vi "Main.vi"() -> ()   [LabVIEW 2016]
uses:
  <vilib>/Instr/_visa.llb/VISA Open Access Mode.ctl
  <vilib>/Instr/_visa.llb/VISA Configure Serial Port (Instr).vi
panel:
  in  "Tab Control":enum32{"Main Program", "Calibration"}(tab)
  in  "Sampling rate (sample/s)":dbl=10.0
  out "Waveform Chart":cluster{u8, u8, u8, u8, u8, u8, u8, u8}(graph)
  in  "Current set (mA)":u16[](array[numeric])
  in  "update curr":bool
  out "Thermometer":i8(slide) scale=10.0..130.0
  out "Temp °C":i8
  in  "VISA resource name":refnum<visa-resource-name>
  in  "relay_1":bool
  in  "relay_2":bool
  in  "relay_3":bool
  in  "relay_4":bool
  in  "relay_5":bool
  in  "relay_6":bool
  in  "relay_7":bool
  out "connected?":bool
  in  "Ch1":bool
  in  "Ch2":bool
  in  "Ch3":bool
  in  "Ch4":bool
  in  "Ch5":bool
  in  "Ch6":bool
  in  "Ch7":bool
  in  "Ch8":bool
  in  "active_ch 1":bool
  in  "active_ch 2":bool
  in  "active_ch 3":bool
  in  "active_ch 4":bool
  in  "active_ch 5":bool
  in  "active_ch 6":bool
  in  "active_ch 7":bool
  in  "active_ch 8":bool
  in  "START":bool
  in  "stop 2":bool
  in  "stop":bool
  out "received voltage data":u8[](array[numeric])
  in  "calib_low":u16[](array[numeric]) max=4095 step=1 format="%03x"
  in  "calib_high":u16[](array[numeric]) max=4095 step=1 format="%03x"
  in  "update_eeprom":bool
  out "eeprom_calib_data":u8[](array[numeric]) format="%02x"
  in  "read_calib":bool
  # "Active \nchannels"
  # "6V max"
  # "16V max"
  # "Relays"
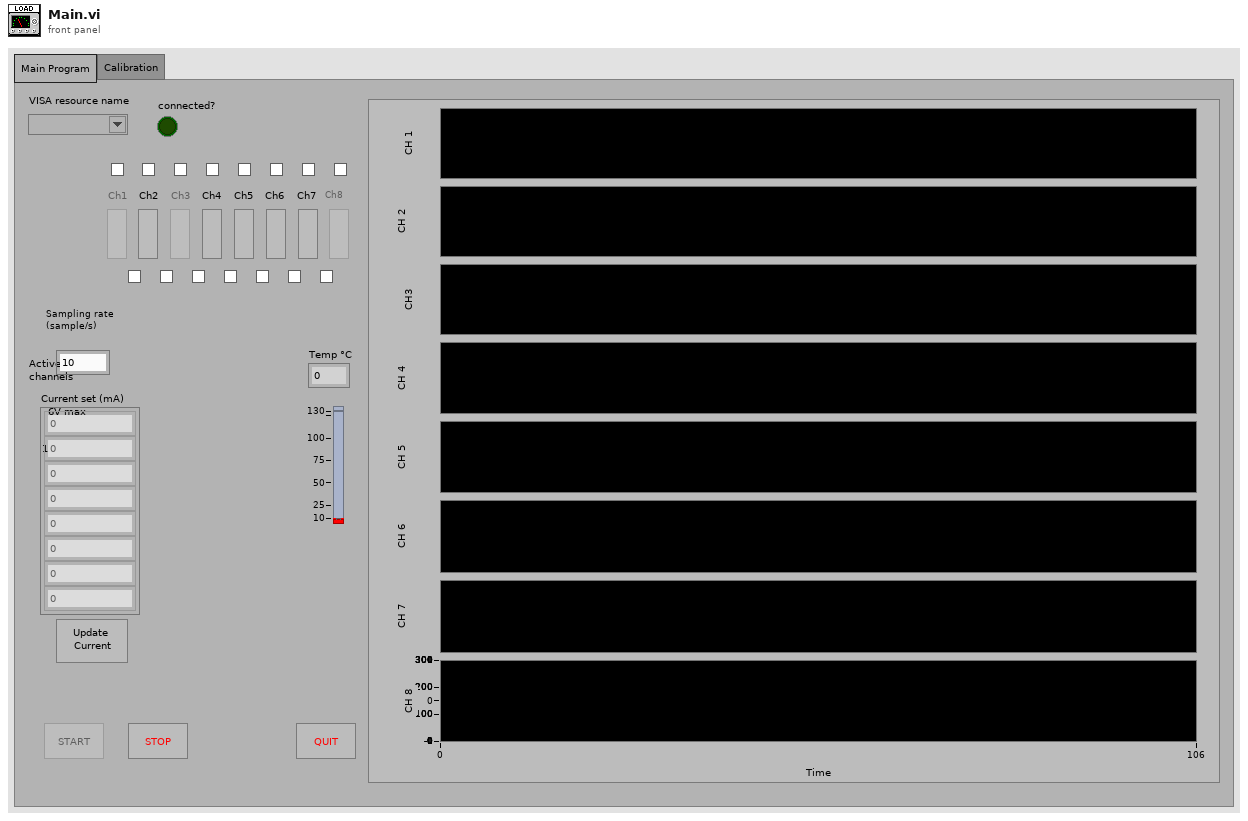
[diagram p1: front panel]
types:
  T1 = enum8{"Enabled", "Disabled", "Disabled and Grayed Out"}
  T2 = typedef "VISA Open Access Mode.ctl" = u32
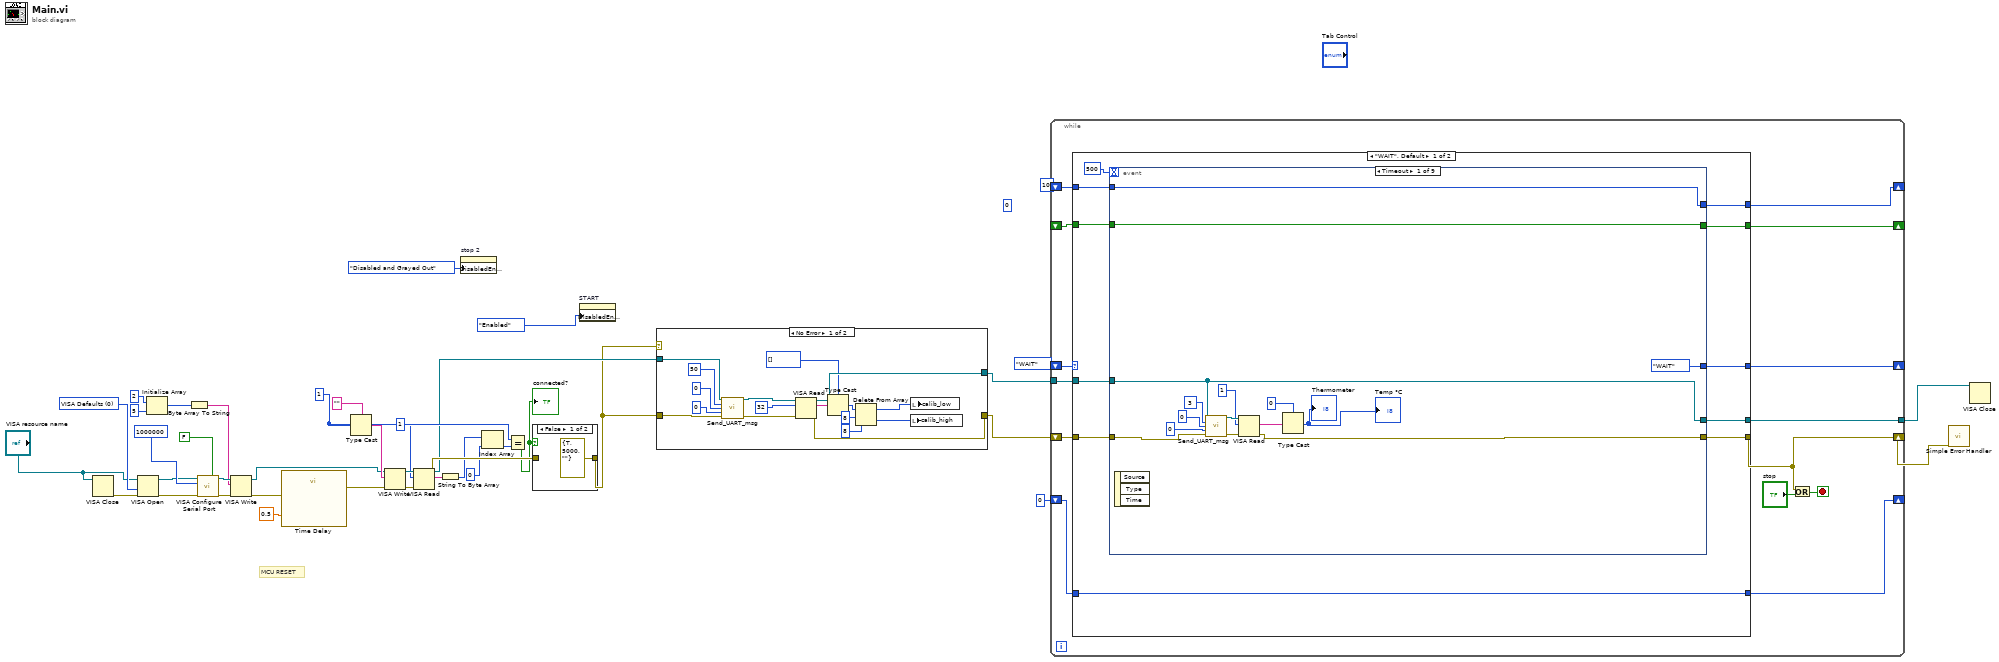
[diagram p0: block diagram]
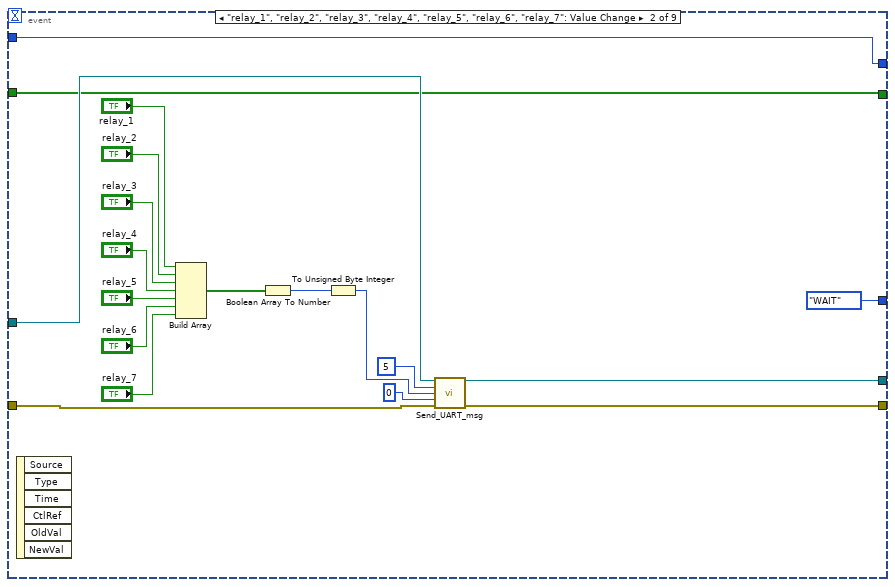
[diagram p3: hidden frame]
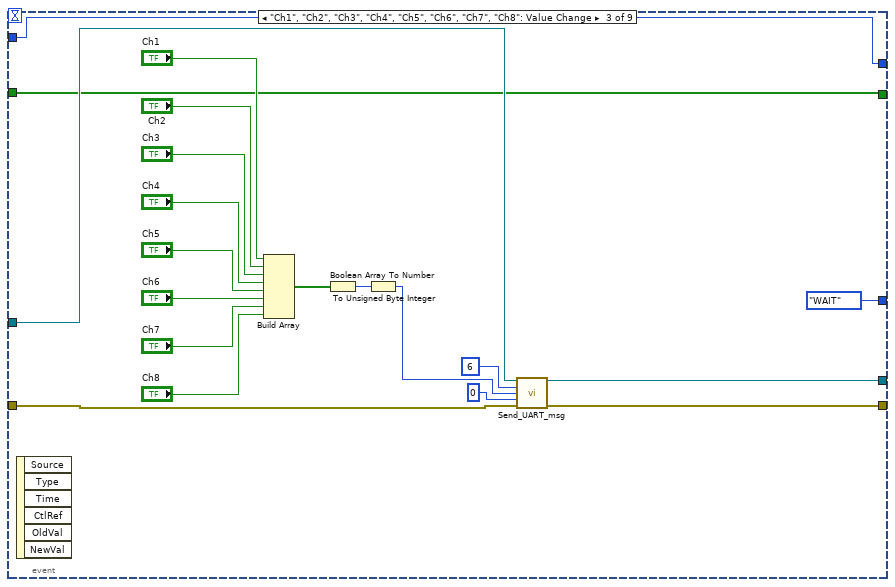
[diagram p4: hidden frame]
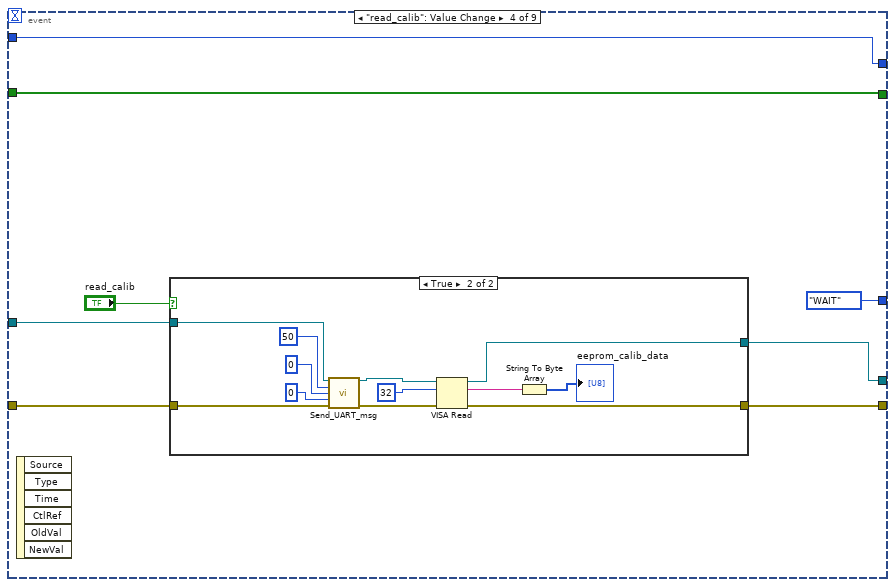
[diagram p5: hidden frame]
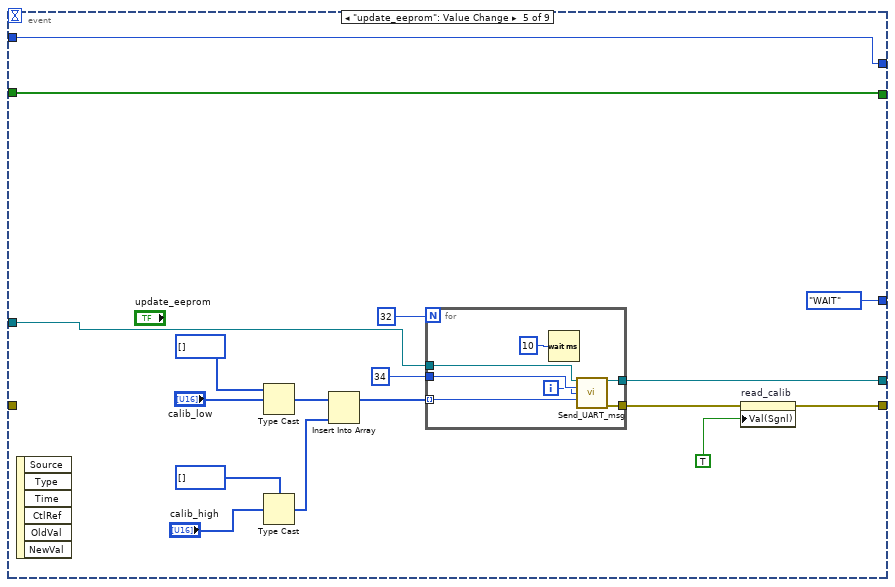
[diagram p7: hidden frame]
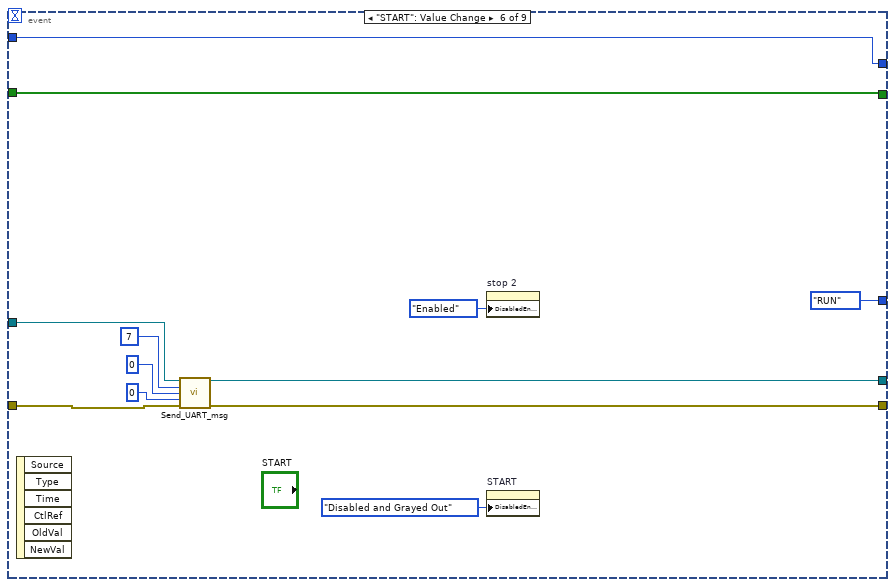
[diagram p8: hidden frame]
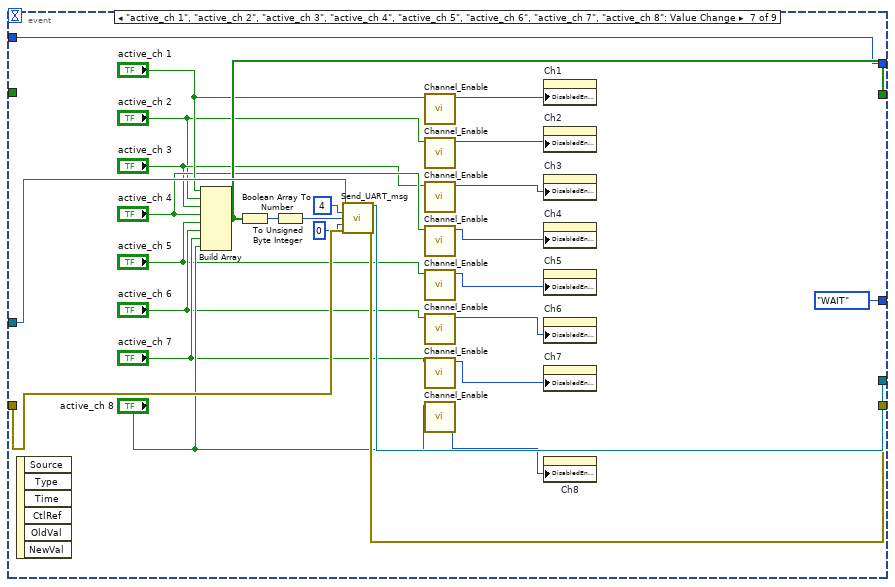
[diagram p9: hidden frame]
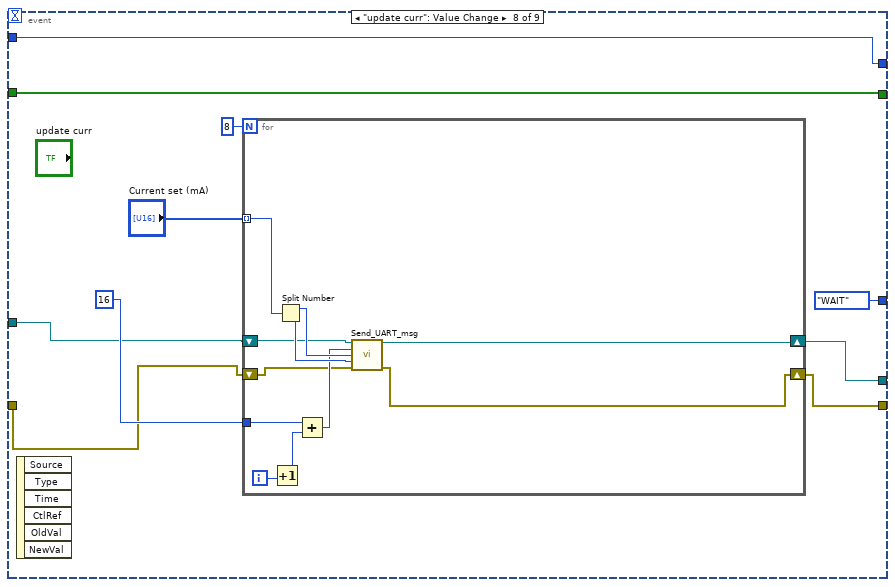
[diagram p10: hidden frame]
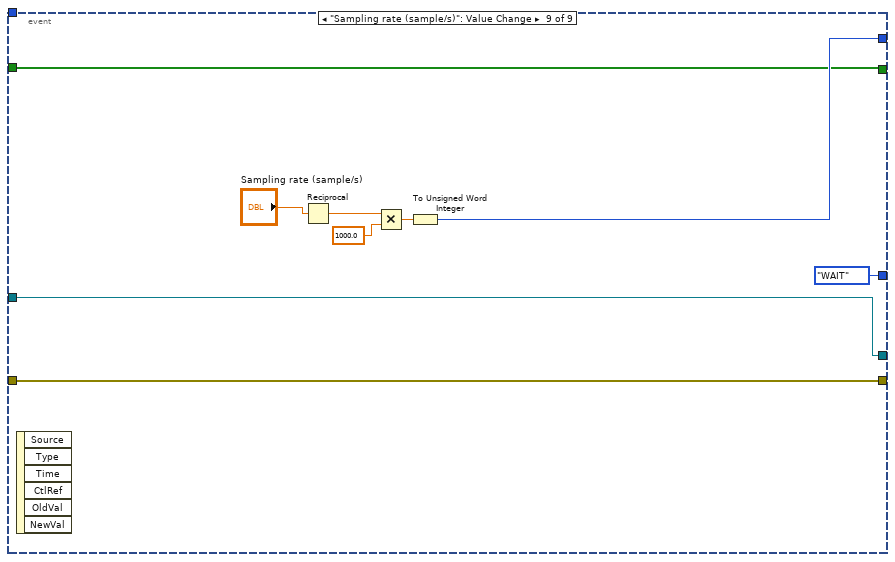
[diagram p11: hidden frame]
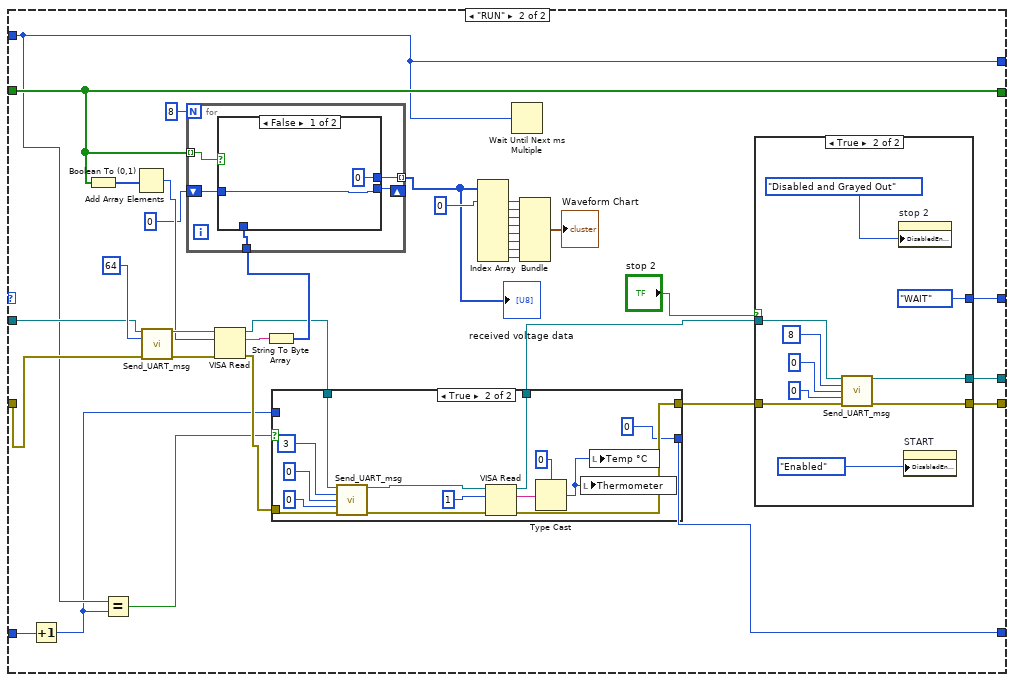
[diagram p12: hidden frame]
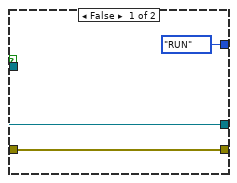
[diagram p14: hidden frame]
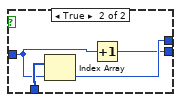
[diagram p15: hidden frame]
diagram:
  (unwired) u8 0
  w23 = T2 0 items=["VISA Defaults"=0, "Exclusive Lock"=1, "Load Configured Settings"=4] ("Access Mode")
  w35 = 1
  # "MCU RESET"
  n1 = VISA Close(VISA resource name="VISA resource name") -> (error out=w20:errorcluster)  [unwired: 1 in]
  n2 = VISA Open(access mode=w23, error in (no error)=w20, VISA resource name="VISA resource name") -> (VISA resource name=w25:refnum<visa-resource-name>, error out=w24:errorcluster)  [unwired: 2 in]
  n3 = Initialize Array(u8 2 ("element"), 5 ("dimension size")) -> (w17:u8[])
  n4 = Byte Array To String(unsigned byte array=w17) -> (string=w14:string)
  n5 = call-poly "VISA Configure Serial Port"("VISA resource name"=w25, "Enable Termination\nChar (T)"=FALSE ("Enable Termination\nChar (T)"), "baud rate (9600)"=u32 1000000, "error in (no error)"=w24) -> ("VISA resource name out"=w15:refnum<visa-resource-name>, "error out"=w16:errorcluster)  [unwired: 10 in]
  n6 = VISA Write(VISA resource name=w15, write buffer=w14, error in (no error)=w16) -> (VISA resource name out=w10:refnum<visa-resource-name>, error out=w12:errorcluster)  [unwired: 1 out]
  n7 = call "Time Delay"("error in (no error)"=w12, "Delay Time (s)"=0.5) -> ("error out"=w11:errorcluster)  [unwired: 9 in]
  n8 = Type Cast(type="", x=w35) -> (*(type *) &x=w40:string)
  n9 = VISA Write(VISA resource name=w10, write buffer=w40, error in (no error)=w11) -> (VISA resource name out=w37:refnum<visa-resource-name>, error out=w36:errorcluster)  [unwired: 1 out]
  n10 = VISA Read(VISA resource name=w37, byte count=u32 1, error in (no error)=w36) -> (VISA resource name out=w5:refnum<visa-resource-name>, read buffer=w30:string, error out=w34:errorcluster)  [unwired: 1 out]
  n11 = String To Byte Array(string=w30) -> (unsigned byte array=w28:u8[])
  n12 = property on="stop 2" class="Bool"("DisabledEnum"=T1."Disabled and Grayed Out" ("Disabled")) -> ()  [unwired: 2 in, 2 out]
  n13 = Index Array(array=w28, index=0) -> (element=w26:u8)
  n14 = Equal?(x=w35, y=w26) -> (x = y?=w29:bool)
  "connected?" <- w29
  n15 = case shown="False" w29 {
    tunnel: [errorcluster {"status"=TRUE, "code"=5000, "source"=""} ("error constant") w42] -> w3
    tunnel: w34 -> [_ w42]
    frame False {
    }
    frame True {
    }
  }
  n16 = property on="START" class="Bool"("DisabledEnum"=T1."Enabled" ("Disabled")) -> ()  [unwired: 2 in, 2 out]
  n17 = case shown="No Error" w3 {
    tunnel: w3 -> [w56 w60]
    tunnel: w5 -> [w55 w61]
    tunnel: [w51 w61] -> w4
    tunnel: [w50 w60] -> w6
    frame No Error {
      n18 = call "Send_UART_msg.vi"("VISA Refnum in"=w55, "Command"=u8 50, "Data 1"=u8 0, "Data 2"=u8 0, "error in (no error)"=w56) -> ("VISA Refnum out"=w53:refnum<visa-resource-name>, "error out"=w54:errorcluster)  [unwired: 8 in, 1 out]
      n19 = VISA Read(VISA resource name=w53, byte count=u32 32, error in (no error)=w54) -> (VISA resource name out=w51:refnum<visa-resource-name>, read buffer=w45:string, error out=w50:errorcluster)  [unwired: 1 out]
      n20 = Type Cast(type=u16[] [], x=w45) -> (*(type *) &x=w44:u16[])
      n21 = Delete From Array(array=w44, length=8, index=8) -> (deleted portion=w47:u16[], array with subset deleted=w46:u16[])
      n22 = local write "calib_high"(w47) -> ()
      n23 = local write "calib_low"(w46) -> ()
    }
    frame Error {
    }
  }
  n24 = while {
    shift-right: [w71] -> w9
    shift-left: w6 -> [w74]
    tunnel: w4 -> [w75]
    shift-right: [w68] -> _
    shift-left: enum16{"WAIT", "RUN", "LOST"}."WAIT" -> [w69]
    tunnel: [w73] -> w22
    shift-right: [w66] -> _
    shift-left: _ -> [w67]
    shift-right: [w65] -> _
    shift-left: u16 10 -> [w64]
    shift-right: [w62] -> _
    shift-left: 0 -> [w63]
    stop <- w70 stop-if-true
    n25 = case shown="\"WAIT\", Default" w69 {
      tunnel: w75 -> [w86 w287]
      tunnel: w74 -> [w85 w286]
      tunnel: [w84 w290] -> w73
      tunnel: [w83 w289] -> w71
      tunnel: [w81 w291] -> w68
      tunnel: w67 -> [w80 w270]
      tunnel: [w79 w270] -> w66
      tunnel: [w78 w263] -> w65
      tunnel: w64 -> [w77 w263]
      tunnel: w63 -> [w76 w264]
      tunnel: [w76 w256] -> w62
      frame "WAIT", Default {
        n26 = event shown="[0] Timeout" {
          selector: _ -> [_ _ _ _ _ _ _ _ _]
          dyn-events: _ -> [_ _ _ _ _ _ _ _ _]
          timeout: 500 -> [_ _ _ _ _ _ _ _ _]
          tunnel: w86 -> [w94 w108 w126 w147 w179 w198 w224 w228 w250]
          tunnel: w85 -> [w101 w106 w129 w148 _ w197 w223 w232 w249]
          tunnel: [w93 w105 w128 w145 w174 w193 w218 w231 w249] -> w83
          tunnel: [w94 w107 w127 w146 w176 w191 w219 w229 w250] -> w84
          tunnel: [enum16{"WAIT", "RUN", "LOST"}."WAIT" enum16{"WAIT", "RUN", "LOST"}."WAIT" enum16{"WAIT", "RUN", "LOST"}."WAIT" enum16{"WAIT", "RUN", "LOST"}."WAIT" enum16{"WAIT", "RUN", "LOST"}."WAIT" enum16{"WAIT", "RUN", "LOST"}."RUN" enum16{"WAIT", "RUN", "LOST"}."WAIT" enum16{"WAIT", "RUN", "LOST"}."WAIT" enum16{"WAIT", "RUN", "LOST"}."WAIT"] -> w81
          tunnel: w80 -> [w91 w103 w122 w142 w164 w188 _ w227 w247]
          tunnel: [w91 w103 w122 w142 w164 w188 w216 w227 w247] -> w79
          tunnel: [w90 w102 w121 w141 w163 w187 w199 w226 w252] -> w78
          tunnel: w77 -> [w90 w102 w121 w141 w163 w187 w199 w226 _]
          event Timeout {
            n27 = event-data() -> ()  [unwired: 1 in, 3 out]
            n28 = call "Send_UART_msg.vi"("VISA Refnum in"=w94, "Command"=u8 3, "Data 1"=u8 0, "Data 2"=u8 0, "error in (no error)"=w101) -> ("VISA Refnum out"=w97:refnum<visa-resource-name>, "error out"=w95:errorcluster)  [unwired: 8 in, 1 out]
            n29 = VISA Read(VISA resource name=w97, byte count=u32 1, error in (no error)=w95) -> (read buffer=w89:string, error out=w93:errorcluster)  [unwired: 2 out]
            n30 = Type Cast(type=i8 0, x=w89) -> (*(type *) &x=→"Thermometer" →"Temp °C":i8)
          }
          event "relay_1", "relay_2", "relay_3", "relay_4", "relay_5", "relay_6", "relay_7": Value Change {
            n31 = event-data() -> ()  [unwired: 1 in, 6 out]
            n32 = Build Array("relay_1", "relay_2", "relay_3", "relay_4", "relay_5", "relay_6", "relay_7") -> (w113:bool[])
            n33 = Boolean Array To Number(Boolean array=w113) -> (number=w112:u32)
            n34 = To Unsigned Byte Integer(number=w112) -> (unsigned 8bit integer=w111:u8)
            n35 = call "Send_UART_msg.vi"("VISA Refnum in"=w108, "Command"=u8 5, "Data 1"=w111, "Data 2"=u8 0, "error in (no error)"=w106) -> ("VISA Refnum out"=w107:refnum<visa-resource-name>, "error out"=w105:errorcluster)  [unwired: 8 in, 1 out]
          }
          event "Ch1", "Ch2", "Ch3", "Ch4", "Ch5", "Ch6", "Ch7", "Ch8": Value Change {
            n36 = event-data() -> ()  [unwired: 1 in, 6 out]
            n37 = Build Array("Ch1", "Ch2", "Ch3", "Ch4", "Ch5", "Ch6", "Ch7", "Ch8") -> (w123:bool[])
            n38 = Boolean Array To Number(Boolean array=w123) -> (number=w132:u32)
            n39 = To Unsigned Byte Integer(number=w132) -> (unsigned 8bit integer=w124:u8)
            n40 = call "Send_UART_msg.vi"("VISA Refnum in"=w126, "Command"=u8 6, "Data 1"=w124, "Data 2"=u8 0, "error in (no error)"=w129) -> ("VISA Refnum out"=w127:refnum<visa-resource-name>, "error out"=w128:errorcluster)  [unwired: 8 in, 1 out]
          }
          event "read_calib": Value Change {
            n41 = event-data() -> ()  [unwired: 1 in, 6 out]
            n42 = case shown="True" "read_calib" {
              tunnel: w148 -> [w149 w159]
              tunnel: w147 -> [w150 w158]
              tunnel: [w150 w154] -> w146
              tunnel: [w149 w153] -> w145
              frame False {
              }
              frame True {
                n43 = call "Send_UART_msg.vi"("VISA Refnum in"=w158, "Command"=u8 50, "Data 1"=u8 0, "Data 2"=u8 0, "error in (no error)"=w159) -> ("VISA Refnum out"=w156:refnum<visa-resource-name>, "error out"=w157:errorcluster)  [unwired: 8 in, 1 out]
                n44 = VISA Read(VISA resource name=w156, byte count=u32 32, error in (no error)=w157) -> (VISA resource name out=w154:refnum<visa-resource-name>, read buffer=w152:string, error out=w153:errorcluster)  [unwired: 1 out]
                n45 = String To Byte Array(string=w152) -> (unsigned byte array=→"eeprom_calib_data":u8[])
              }
            }
          }
          event "update_eeprom": Value Change {
            n46 = event-data() -> ()  [unwired: 1 in, 6 out]
            n47 = Type Cast(type=u8[] [], x="calib_low") -> (*(type *) &x=w168:u8[])
            n48 = Type Cast(type=u8[] [], x="calib_high") -> (*(type *) &x=w167:u8[])
            n49 = Insert Into Array(array=w168, new element=w167) -> (w169:u8[])  [unwired: 1 in]
            n50 = for {
              N: 32 -> [_]
              tunnel: w179 -> [w186]
              tunnel: u8 34 -> [w185]
              tunnel: w169 -> [w183] mode=indexing
              tunnel: [w182] -> w176
              tunnel: [w181] -> w175
              i -> [w184]
              n51 = Wait (ms)(milliseconds to wait=u32 10 ("millisecond multiple")) -> ()  [unwired: 1 out]
              n52 = call "Send_UART_msg.vi"("VISA Refnum in"=w186, "Command"=w185, "Data 1"=w184, "Data 2"=w183) -> ("VISA Refnum out"=w182:refnum<visa-resource-name>, "error out"=w181:errorcluster)  [unwired: 9 in, 1 out]
            }
            n53 = property on="read_calib" class="Bool (strict)"(error in=w175, "Val(Sgnl)"=TRUE ("Value (Signaling)")) -> (error out=w174:errorcluster)  [unwired: 1 in, 1 out]
          }
          event "START": Value Change {
            n54 = event-data() -> ()  [unwired: 1 in, 6 out]
            n55 = call "Send_UART_msg.vi"("VISA Refnum in"=w198, "Command"=u8 7, "Data 1"=u8 0, "Data 2"=u8 0, "error in (no error)"=w197) -> ("VISA Refnum out"=w191:refnum<visa-resource-name>, "error out"=w193:errorcluster)  [unwired: 8 in, 1 out]
            n56 = property on="stop 2" class="Bool"("DisabledEnum"=T1."Enabled" ("Disabled")) -> ()  [unwired: 2 in, 2 out]
            n57 = property on="START" class="Bool"("DisabledEnum"=T1."Disabled and Grayed Out" ("Disabled")) -> ()  [unwired: 2 in, 2 out]
          }
          event "active_ch 1", "active_ch 2", "active_ch 3", "active_ch 4", "active_ch 5", "active_ch 6", "active_ch 7", "active_ch 8": Value Change {
            n58 = event-data() -> ()  [unwired: 1 in, 6 out]
            n59 = Build Array("active_ch 1", "active_ch 2", "active_ch 3", "active_ch 4", "active_ch 5", "active_ch 6", "active_ch 7", "active_ch 8") -> (w216:bool[])
            n60 = Boolean Array To Number(Boolean array=w216) -> (number=w225:u32)
            n61 = To Unsigned Byte Integer(number=w225) -> (unsigned 8bit integer=w222:u8)
            n62 = call "Send_UART_msg.vi"("VISA Refnum in"=w224, "Command"=u8 4, "Data 1"=w222, "Data 2"=u8 0, "error in (no error)"=w223) -> ("VISA Refnum out"=w219:refnum<visa-resource-name>, "error out"=w218:errorcluster)  [unwired: 8 in, 1 out]
            n63 = call "Channel_Enable.vi"("active_ch 1"="active_ch 1") -> ("Disabled"=w215:T1)  [unwired: 10 in]
            n64 = call "Channel_Enable.vi"("active_ch 1"="active_ch 2") -> ("Disabled"=w213:T1)  [unwired: 10 in]
            n65 = call "Channel_Enable.vi"("active_ch 1"="active_ch 3") -> ("Disabled"=w212:T1)  [unwired: 10 in]
            n66 = call "Channel_Enable.vi"("active_ch 1"="active_ch 4") -> ("Disabled"=w211:T1)  [unwired: 10 in]
            n67 = call "Channel_Enable.vi"("active_ch 1"="active_ch 5") -> ("Disabled"=w210:T1)  [unwired: 10 in]
            n68 = call "Channel_Enable.vi"("active_ch 1"="active_ch 6") -> ("Disabled"=w209:T1)  [unwired: 10 in]
            n69 = call "Channel_Enable.vi"("active_ch 1"="active_ch 7") -> ("Disabled"=w208:T1)  [unwired: 10 in]
            n70 = call "Channel_Enable.vi"("active_ch 1"="active_ch 8") -> ("Disabled"=w207:T1)  [unwired: 10 in]
            n71 = property on="Ch1" class="Bool (strict)"("DisabledEnum"=w215) -> ()  [unwired: 2 in, 2 out]
            n72 = property on="Ch2" class="Bool (strict)"("DisabledEnum"=w213) -> ()  [unwired: 2 in, 2 out]
            n73 = property on="Ch3" class="Bool (strict)"("DisabledEnum"=w212) -> ()  [unwired: 2 in, 2 out]
            n74 = property on="Ch4" class="Bool (strict)"("DisabledEnum"=w211) -> ()  [unwired: 2 in, 2 out]
            n75 = property on="Ch5" class="Bool (strict)"("DisabledEnum"=w210) -> ()  [unwired: 2 in, 2 out]
            n76 = property on="Ch6" class="Bool (strict)"("DisabledEnum"=w209) -> ()  [unwired: 2 in, 2 out]
            n77 = property on="Ch7" class="Bool (strict)"("DisabledEnum"=w208) -> ()  [unwired: 2 in, 2 out]
            n78 = property on="Ch8" class="Bool (strict)"("DisabledEnum"=w207) -> ()  [unwired: 2 in, 2 out]
          }
          event "update curr": Value Change {
            n79 = event-data() -> ()  [unwired: 1 in, 6 out]
            n80 = for {
              N: 8 -> [_]
              tunnel: "Current set (mA)" -> [w246] mode=indexing
              tunnel: u8 16 ("Command") -> [w241]
              shift-right: [w239] -> w231
              shift-left: w232 -> [w238]
              shift-right: [w237] -> w229
              shift-left: w228 -> [w236]
              i -> [w243]
              n81 = Increment(x=w243) -> (x+1=w242:i32)
              n82 = Split Number(x=w246) -> (hi(x)=w245:u8, lo(x)=w244:u8)
              n83 = Add(x=w241, y=w242) -> (x+y=w240:i32)
              n84 = call "Send_UART_msg.vi"("VISA Refnum in"=w236, "Command"=w240, "Data 1"=w245, "Data 2"=w244, "error in (no error)"=w238) -> ("VISA Refnum out"=w237:refnum<visa-resource-name>, "error out"=w239:errorcluster)  [unwired: 8 in, 1 out]
            }
          }
          event "Sampling rate (sample/s)": Value Change {
            n85 = event-data() -> ()  [unwired: 1 in, 6 out]
            n86 = Reciprocal(x="Sampling rate (sample/s)") -> (1/x=w251:dbl)
            n87 = Multiply(x=w251, y=1000.0) -> (x*y=w253:dbl)
            n88 = To Unsigned Word Integer(number=w253) -> (unsigned 16bit integer=w252:u16)
          }
        }
      }
      frame "RUN" {
        n89 = Increment(x=w264) -> (x+1=w257:i32)
        n90 = Boolean To (0,1)(Boolean=w270) -> (0, 1=w283:i16[])
        n91 = Equal?(x=w263, y=w257) -> (x = y?=w261:bool)
        n92 = Add Array Elements(numeric array=w283) -> (sum=w282:i16)
        n93 = call "Send_UART_msg.vi"("VISA Refnum in"=w287, "Command"=u8 64, "error in (no error)"=w286) -> ("VISA Refnum out"=w285:refnum<visa-resource-name>, "error out"=w284:errorcluster)  [unwired: 10 in, 1 out]
        n94 = VISA Read(VISA resource name=w285, byte count=w282, error in (no error)=w284) -> (VISA resource name out=w260:refnum<visa-resource-name>, read buffer=w281:string, error out=w262:errorcluster)  [unwired: 1 out]
        n95 = String To Byte Array(string=w281) -> (unsigned byte array=w269:u8[])
        n96 = for {
          N: 8 -> [_]
          tunnel: w270 -> [w326] mode=indexing
          tunnel: w269 -> [w323]
          tunnel: [w325] -> w266 mode=indexing
          shift-right: [w322] -> _
          shift-left: 0 -> [w324]
          n97 = case shown="False" w326 {
            tunnel: [u8 0 w331] -> w325
            tunnel: w324 -> [w327 w329]
            tunnel: w323 -> [_ w332]
            tunnel: [w327 w330] -> w322
            frame False {
            }
            frame True {
              n98 = Index Array(array=w332, index=w329) -> (element=w331:u8)
              n99 = Increment(x=w329) -> (x+1=w330:i32)
            }
          }
        }
        "received voltage data" <- w266
        n100 = case shown="True" w261 {
          tunnel: w262 -> [w293 w301]
          tunnel: w260 -> [w294 w300]
          tunnel: [w294 w299] -> w259
          tunnel: [w293 w296] -> w258
          tunnel: w257 -> [w292 _]
          tunnel: [w292 0] -> w256
          frame False {
          }
          frame True {
            n101 = call "Send_UART_msg.vi"("VISA Refnum in"=w300, "Command"=u8 3, "Data 1"=u8 0, "Data 2"=u8 0, "error in (no error)"=w301) -> ("VISA Refnum out"=w305:refnum<visa-resource-name>, "error out"=w303:errorcluster)  [unwired: 8 in, 1 out]
            n102 = VISA Read(VISA resource name=w305, byte count=u32 1, error in (no error)=w303) -> (VISA resource name out=w299:refnum<visa-resource-name>, read buffer=w302:string, error out=w296:errorcluster)  [unwired: 1 out]
            n103 = Type Cast(type=u8 0, x=w302) -> (*(type *) &x=w297:u8)
            n104 = local write "Thermometer"(w297) -> ()
            n105 = local write "Temp °C"(w297) -> ()
          }
        }
        n106 = Index Array(array=w266, index #1=0 ("index")) -> (element #1=w272:u8, element #2=w273:u8, element #3=w274:u8, element #4=w275:u8, element #5=w276:u8, element #6=w277:u8, element #7=w278:u8, element #8=w279:u8)  [unwired: 7 in]
        n107 = Wait Until Next ms Multiple(millisecond multiple=w263) -> ()  [unwired: 1 out]
        n108 = Bundle(w272, w273, w274, w275, w276, w277, w278, w279) -> (→"Waveform Chart":cluster{u8, u8, u8, u8, u8, u8, u8, u8})  [unwired: 1 in]
        n109 = case shown="True" "stop 2" {
          tunnel: [enum16{"WAIT", "RUN", "LOST"}."RUN" enum16{"WAIT", "RUN", "LOST"}."WAIT"] -> w291
          tunnel: [w310 w320] -> w290
          tunnel: [w309 w319] -> w289
          tunnel: w258 -> [w309 w318]
          tunnel: w259 -> [w310 w317]
          frame False {
          }
          frame True {
            n110 = call "Send_UART_msg.vi"("VISA Refnum in"=w317, "Command"=u8 8, "Data 1"=u8 0, "Data 2"=u8 0, "error in (no error)"=w318) -> ("VISA Refnum out"=w320:refnum<visa-resource-name>, "error out"=w319:errorcluster)  [unwired: 8 in, 1 out]
            n111 = property on="stop 2" class="Bool"("DisabledEnum"=T1."Disabled and Grayed Out" ("Disabled")) -> ()  [unwired: 2 in, 2 out]
            n112 = property on="START" class="Bool"("DisabledEnum"=T1."Enabled" ("Disabled")) -> ()  [unwired: 2 in, 2 out]
          }
        }
      }
    }
    n113 = Or(x=w71, y="stop") -> (x .or. y?=w70:bool)
  }
  n114 = call <vilib>:"Simple Error Handler.vi"("error in (no error)"=w9) -> ()  [unwired: 4 in, 5 out]
  n115 = VISA Close(VISA resource name=w22) -> ()  [unwired: 1 in, 1 out]
